vi "Component.vi"(6 "Teller":refnum<class "Teller.lvclass">, 7 "Actor in":refnum<class "Actor.lvclass">) -> (0 "Error out":errorcluster, 5 "Actor out":refnum<class "Actor.lvclass">)   [LabVIEW 2025, in "_Template.lvlib" / "Templates.lvlib" / "TEMPLATE Msg.lvlib"]
uses:
  TEMPLATE Msg.lvlib
  jettl/jettl/Actor/Actor/Actor.lvclass
  jettl/jettl/Teller/Teller/Teller.lvclass
  TEMPLATE Msg/TEMPLATE Msg.lvclass
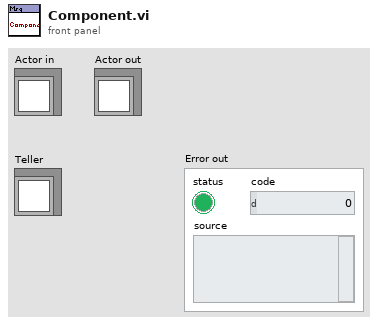
[diagram p1: front panel]
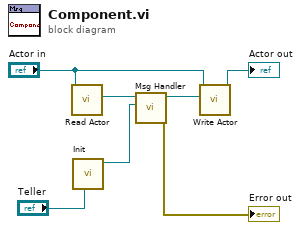
[diagram p0: block diagram]
diagram:
  n1 = call-dynamic "Read Actor.vi"("Actor in"="Actor in") -> ("Actor"=w6:refnum<class "Actor.lvclass">)  [unwired: 10 in]
  n2 = call "Init.vi"("Teller"="Teller") -> ("TEMPLATE Msg out"=w3:refnum<class "TEMPLATE Msg.lvclass">)  [unwired: 10 in]
  n3 = call-dynamic "Msg Handler.vi"("Msg"=w3, "Actor in"=w6) -> ("Error out"=→"Error out":errorcluster, "Actor out"=w5:refnum<class "Actor.lvclass">)  [unwired: 8 in]
  n4 = call-dynamic "Write Actor.vi"("Actor"=w5, "Actor in"="Actor in") -> ("Actor out"=→"Actor out":refnum<class "Actor.lvclass">)  [unwired: 9 in]
